vi "Send Event with Logging.vi"(4 "Global Log Level":T1, 6 "Message Priority":T2, 7 "Mediated Actor in":refnum<class "Mediated Actor.lvclass">, 8 "error in (no error)":errorcluster, 9 "Timeout":i32, 10 "Message":refnum<class "Message Interface.lvclass">, 11 "Message Transport Interface in":refnum<class "Message Transport Interface.lvclass">) -> (0 "error out":errorcluster, 5 "Mediated Actor out":refnum<class "Mediated Actor.lvclass">)   [LabVIEW 2016, in "Stream Mediator.lvlib" / "Mediated Actor.lvclass"]
doc: "--\nCopyright © 2017 Composed SystemsI All rights reserved.\n\nAuthor: Jon McBee <jon.mcbee@composed.io>\n\nThis library is provided \"AS IS\" ,WITHOUT WARRANTIES OR\nCONDITIONS OF ANY KIND, either express or implied.\n\nComposed Systems -- composed.io\n\nStream 0.0.1.1\nJon McBee - Composed Systems\nCopyright (c) 2017, Composed Systems"
uses:
  <userlib>/Composed Systems/Stream/Mediator/Classes/Mediated Actor/Mediated Actor.lvclass
  C:/Program Files (x86)/National Instruments/LabVIEW 2016/user.lib/Composed Systems/Stream/Actor/Actor Class/Ancestral Actor.lvclass
  <userlib>/Composed Systems/Stream/Mediator/Classes/Message Interface/Message Interface.lvclass
  <userlib>/Composed Systems/Stream/Mediator/Classes/Message Transport Interface/Message Transport Interface.lvclass
  <userlib>/Composed Systems/Stream/Mediator/Classes/Message Transport Interface/Message Priority.ctl
  <userlib>/Composed Systems/Stream/Log/Application Log/Log Level.ctl
  <userlib>/Composed Systems/Stream/Actor/Actor Class/Ancestral Actor.lvclass/Ancestral Actor.ctl
  <userlib>/Composed Systems/Stream/Log/Global Application Log/Global Application Log.lvclass
  <userlib>/Composed Systems/Stream/Actor/Actor Class/Ancestral Actor.lvclass
  <userlib>/Composed Systems/Stream/Log/Application Log/Application Log.lvclass
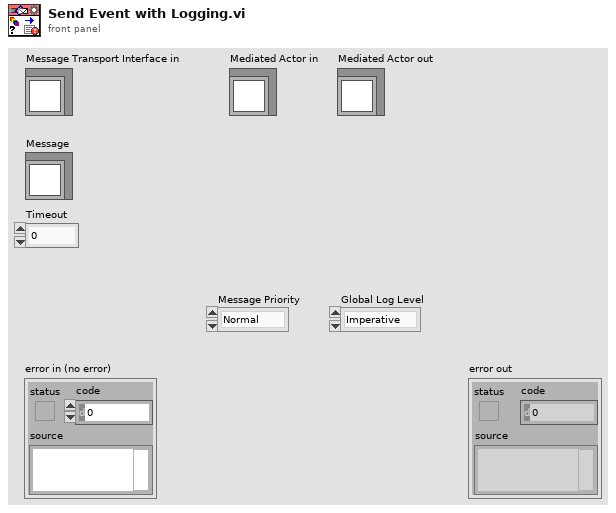
[diagram p1: front panel]
types:
  T1 = typedef "Stream Log.lvlib/Application Log.lvclass/Log Level.ctl" = enum16{"Imperative", "Major", "Minor", "Debug", "Off"}
  T2 = typedef "Stream Mediator.lvlib/Message Transport Interface.lvclass/Message Priority.ctl" = enum16{"Normal", "High"}
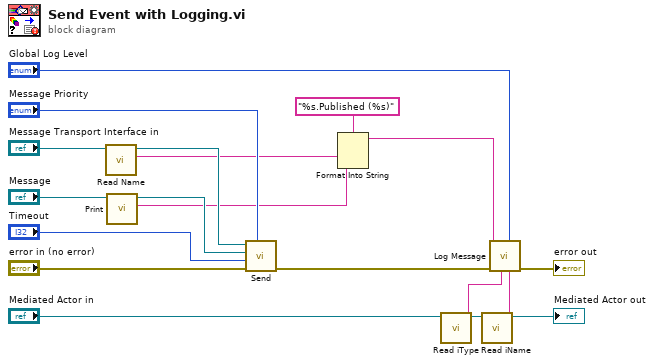
[diagram p0: block diagram]
diagram:
  n1 = call <userlib>:"Read Name.vi"("Message Transport Interface in"="Message Transport Interface in") -> ("Name"=w2:string, "Message Transport Interface out"=w3:refnum<class "Message Transport Interface.lvclass">)  [unwired: 8 in, 1 out]
  n2 = call-dynamic "Print.vi"("Message Interface in"="Message") -> ("String"=w1:string, "Message Interface out"=w7:refnum<class "Message Interface.lvclass">)  [unwired: 8 in, 1 out]
  n3 = call-dynamic "Send.vi"("Message Priority"="Message Priority", "error in (no error)"="error in (no error)", "Timeout"="Timeout", "Message"=w7, "Message Transport Interface in"=w3) -> ("error out"=w15:errorcluster)  [unwired: 4 in, 2 out]
  n4 = Format Into String(format string="%s.Published (%s)", w2, w1) -> (resulting string=w5:string)  [unwired: 2 in, 1 out]
  n5 = call <userlib>:"Read iType.vi"("Ancestral Actor in"="Mediated Actor in") -> ("iType"=w10:string, "Ancestral Actor out"=w12:refnum<class "Mediated Actor.lvclass">)  [unwired: 8 in, 1 out]
  n6 = call <userlib>:"Read iName.vi"("Ancestral Actor in"=w12) -> ("iName"=w9:string, "Ancestral Actor out"=→"Mediated Actor out":refnum<class "Mediated Actor.lvclass">)  [unwired: 8 in, 1 out]
  n7 = call <userlib>:"Log Message.vi"("Actor Name"=w9, "Level"="Global Log Level", "Actor Type"=w10, "error in (no error)"=w15, "Message"=w5) -> ("error out"=→"error out":errorcluster)  [unwired: 6 in]
